vi "Get Array of Conflict Zones.vi"(8 "error in (no error)":errorcluster, 11 "VacuumLines Configuration in":refnum<class "VacuumLines Configuration.lvclass">) -> (0 "error out":errorcluster, 2 "Array of Conflict Zones":T1[](array[typedef]) caption="Conflict Zones (unit in mm)", 3 "VacuumLines Configuration out":refnum<class "VacuumLines Configuration.lvclass">)   [LabVIEW 2016, in "Hardware.lvlib" / "VacuumLine.lvlib" / "VacuumLines Configuration.lvclass"]
uses:
  <userlib>/Common Components/Hardware/Abstract System/VacuumLine/VacuumLines Configuration/VacuumLines Configuration.lvclass
  <userlib>/Common Components/Hardware/Abstract System/VacuumLine/VacuumLines/Conflict Zone.ctl
  <userlib>/Common Components/Hardware/Abstract System/VacuumLine/VacuumLines Configuration/VacuumLines Configuration.lvclass/VacuumLines Configuration.ctl
  <userlib>/Common Components/Hardware/Abstract System/VacuumLine/VacuumLines/VacuumLines.lvclass/VacuumLines.ctl
  <userlib>/Common Components/Hardware/Abstract System/VacuumLine/VacuumLines/VacuumLines.lvclass
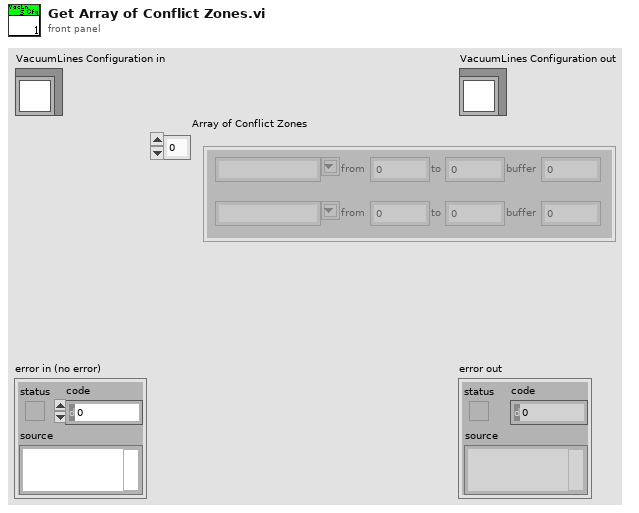
[diagram p1: front panel]
types:
  T1 = typedef "Hardware.lvlib/VacuumLine.lvlib/VacuumLines.lvclass/Conflict Zone.ctl" = cluster{"Conflict Zone":cluster{"1":cluster{"Label":string, "from":dbl, "to":dbl, "buffer":dbl}, "2":cluster{"Label":string, "from":dbl, "to":dbl, "buffer":dbl}}}
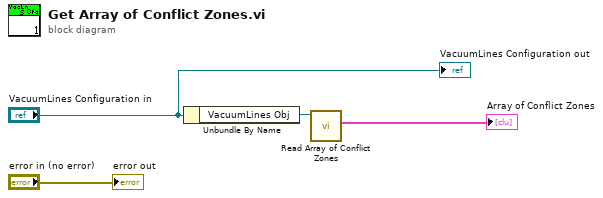
[diagram p0: block diagram]
diagram:
  n1 = Unbundle By Name("VacuumLines Configuration in") -> ("VacuumLines Obj"=w2:refnum<class "VacuumLines.lvclass">)
  n2 = call <userlib>:"Read Array of Conflict Zones.vi"("VacuumLines in"=w2) -> ("Array of Conflict Zones"=→"Array of Conflict Zones":T1[])  [unwired: 9 in, 1 out]
  "error out" <- "error in (no error)"
  "VacuumLines Configuration out" <- "VacuumLines Configuration in"
